vi "LD2018_ブロック崩し_ブロック範囲.vi"(2 "長さ/幅":i32, 3 "直前エリア位置":i32) -> (0 "最大値":i32, 1 "最小値":i32)   [LabVIEW 2017]
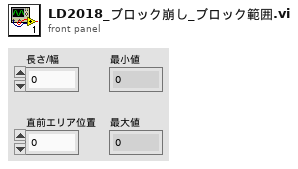
[diagram p1: front panel]
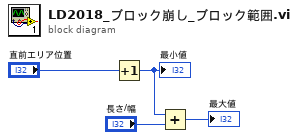
[diagram p0: block diagram]
diagram:
  n1 = Increment(x="直前エリア位置") -> (x+1=w2:i32)
  "最小値" <- w2
  n2 = Add(x=w2, y="長さ/幅") -> (x+y=→"最大値":i32)
